vi "emi_Anything Changed.vi"(7 "Anything":variant) -> (8 "changed":bool)   [LabVIEW 2010]
doc: "Compares any value with its previous value.\n\nFirst call will always give a false output\n\nUses variant, will except anything, note: Slow with large sets.\nDedicated type comparison will always be faster.\n\nreentrant Subroutine."
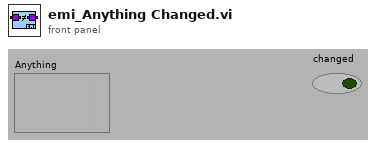
[diagram p1: front panel]
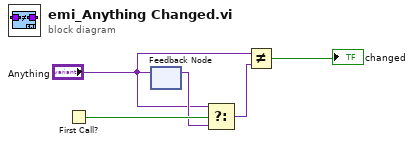
[diagram p0: block diagram]
diagram:
  n1 = First Call?() -> (First Call?: T/F=w5:bool)
  n2 = feedback-in #1("Anything") -> ()
  n3 = feedback #1() -> (w4:variant)  [unwired: 1 in]
  n4 = Select(t="Anything", s=w5, f=w4) -> (s? t:f=w3:variant)
  n5 = Not Equal?(x="Anything", y=w3) -> (x != y?=→"changed":bool)
